vi "E364XA Commands SA 2.vi"(0 "VISA session":refnum<visa-resource-name>="COM3", 1 "Voltage":string, 7 "Command":u16(ring) items=["Output Off", "Output On", "Output?", "Voltage Range Low", "Voltage Range High", "Voltage Range?", "Apply 12V, 1.5A", "Apply?", "Voltage 12V", "Voltage?", "Current 1.5A", "Current?", "Measure Voltage", "Measure Current", "Set RS232", "Set Remote Mode", "Set Local Mode", "System Error?", "*IDN?", "*RST", "Instrument Sel?", "Instrument Sel Out 1", "Instrument Sel Out 2", "Display Mode VI", "Display Mode VV", "Display Mode II", "Apply 0V, 0A", "Set Voltage"], 11 "error in (no error)":errorcluster) -> (4 "VISA session out":refnum<visa-resource-name>, 6 "Response":string, 8 "Num Resp":dbl, 13 "Bytes at port":u8, 14 "Bytes Read":u8, 15 "error out":errorcluster)   [LabVIEW 2010]
uses:
  <vilib>/Instr/_visa.llb/VISA Configure Serial Port (Instr).vi
panel:
  in  "Serial Configuration":T1={"Baud Rate"=9600, "Parity"=0, "Data Bits"=8, "Stop Bits"=20, "Flow Control"=0} {"Flow Control" items=["None", "XON/XOFF", "RTS/CTS", "XON/XOFF & RTS/CTS", "DTR/DSR", "XON/XOFF & DTR/DSR"]; "Stop Bits" items=["1.0"=10, "1.5"=15, "2.0"=20]; "Data Bits" items=["7"=7, "8"=8]; "Parity" items=["None", "Odd", "Even", "Mark", "Space"]; "Baud Rate" items=["300"=300, "600"=600, "1200"=1200, "2400"=2400, "4800"=4800, "9600"=9600, "19200"=19200]}
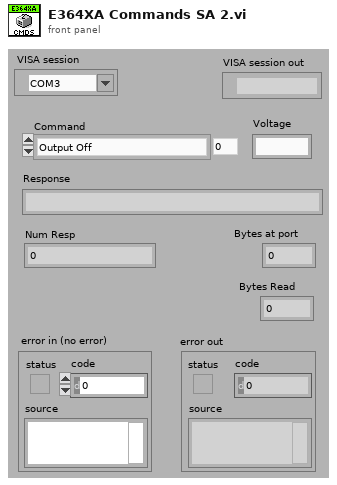
[diagram p1: front panel]
types:
  T1 = cluster{"Baud Rate":u32, "Parity":u16, "Data Bits":u16, "Stop Bits":u16, "Flow Control":u16}
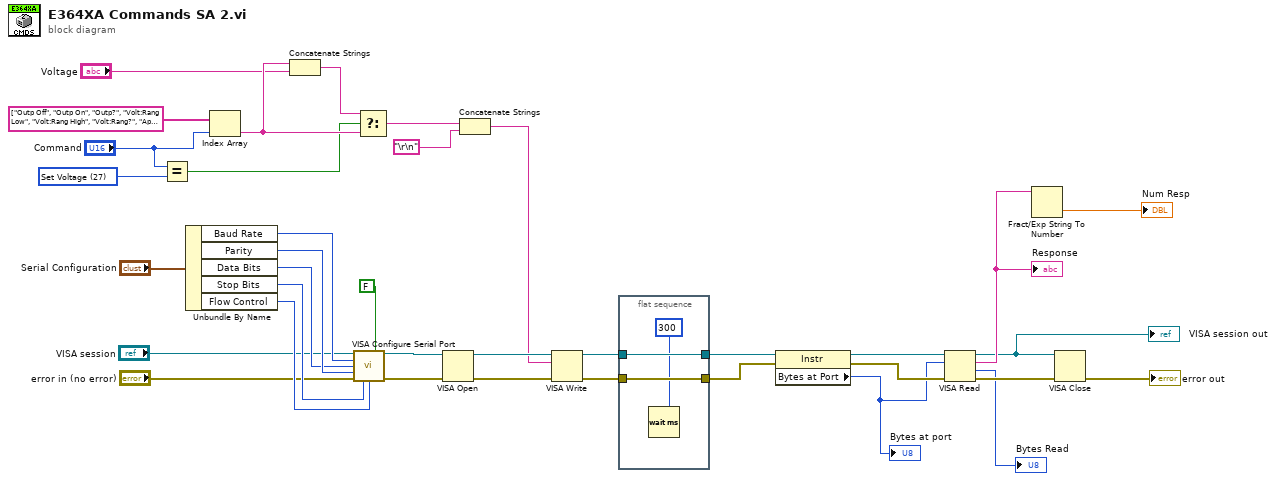
[diagram p0: block diagram]
diagram:
  w6 = u16 27 items=["Output Off", "Output On", "Output?", "Voltage Range Low", "Voltage Range High", "Voltage Range?", "Apply 12V, 1.5A", "Apply?", "Voltage 12V", "Voltage?", "Current 1.5A", "Current?", "Measure Voltage", "Measure Current", "Set RS232", "Set Remote Mode", "Set Local Mode", "System Error?", "*IDN?", "*RST", "Instrument Sel?", "Instrument Sel Out 1", "Instrument Sel Out 2", "Display Mode VI", "Display Mode VV", "Display Mode II", "Apply 0V, 0A", "Set Voltage"] ("Command")
  n1 = Equal?(x="Command", y=w6) -> (x = y?=w3:bool)
  n2 = Unbundle By Name("Serial Configuration") -> ("Baud Rate"=w35:u32, "Parity"=w34:u16, "Data Bits"=w33:u16, "Stop Bits"=w32:u16, "Flow Control"=w31:u16)
  n3 = Index Array(array=string[] ["Outp Off", "Outp On", "Outp?", "Volt:Rang Low", "Volt:Rang High", "Volt:Rang?", "Apply 12,1.5", "Apply?", "Volt 12", "Volt?", "Curr 1.5", "Curr?", "Meas:Volt?", "Meas:curr?", "Syst:Int RS232", "Syst:Rem", "Syst:Loc", "Syst:Err?", "*IDN?", "*RST", "INST:SEL?", "INST:SEL OUT1", "INST:SEL OUT2", "DISP:MODE VI", "DISP:MODE VV", "DISP:MODE II", "Apply 0,0", "Volt "], index="Command") -> (element=w4:string)
  n4 = Concatenate Strings(w4, "Voltage") -> (w1:string)
  n5 = call-poly "VISA Configure Serial Port"("VISA resource name"="VISA session", "Enable Termination\nChar (T)"=FALSE, "baud rate (9600)"=w35, "data bits (8)"=w33, "parity (0:none)"=w34, "error in (no error)"="error in (no error)", "stop bits (10: 1 bit)"=w32, "flow control (0:none)"=w31) -> ("VISA resource name out"=w27:refnum<visa-resource-name>, "error out"=w26:errorcluster)  [unwired: 6 in]
  n6 = Select(t=w1, s=w3, f=w4) -> (s? t:f=w5:string)
  n7 = VISA Open(error in (no error)=w26, VISA resource name=w27) -> (VISA resource name=w24:refnum<visa-resource-name>, error out=w25:errorcluster)  [unwired: 3 in]
  n8 = Concatenate Strings(w5, "\r\n") -> (w22:string)
  n9 = VISA Write(VISA resource name=w24, write buffer=w22, error in (no error)=w25) -> (VISA resource name out=w15:refnum<visa-resource-name>, error out=w14:errorcluster)  [unwired: 1 out]
  n10 = flat-sequence {
    tunnel: [w39] -> w12
    tunnel: w15 -> [w39]
    tunnel: [w38] -> w13
    tunnel: w14 -> [w38]
    frame #0 {
      n11 = Wait (ms)(milliseconds to wait=300) -> ()  [unwired: 1 out]
    }
  }
  n12 = property class="Instr"(reference=w12, error in=w13) -> (reference out=w18:refnum<visa-resource-name>, error out=w17:errorcluster, "Bytes at Port"=w16:u32)
  "Bytes at port" <- w16
  n13 = VISA Read(VISA resource name=w18, byte count=w16, error in (no error)=w17) -> (VISA resource name out=w8:refnum<visa-resource-name>, read buffer=w11:string, return count=→"Bytes Read":u32, error out=w20:errorcluster)
  "Response" <- w11
  "VISA session out" <- w8
  n14 = Fract/Exp String To Number(string=w11) -> (number=→"Num Resp":dbl)  [unwired: 3 in, 1 out]
  n15 = VISA Close(VISA resource name=w8, error in (no error)=w20) -> (error out=→"error out":errorcluster)
